vi "svx_Set Limits Interactively.vi"(7 "move upper or lower limit together":bool, 8 "error in":errorcluster, 10 "limits in":dbl[](array[numeric])=[0.0, 0.0, 0.0, 0.0, 0.0, 0.0, 0.0, 0.0, 0.0, 0.0, 0.0, 0.0, 0.0, 0.0, 0.0, 0.0, 0.0, 0.0, 0.0, 0.0], 11 "limit graph control refnum":refnum<vi>) -> (0 "error out":errorcluster, 2 "limits out":dbl[](array[numeric]), 3 "dup limit graph control refnum":refnum<vi>)   [LabVIEW 2017]
panel:
  out "limits graph":dbl[][](graph)
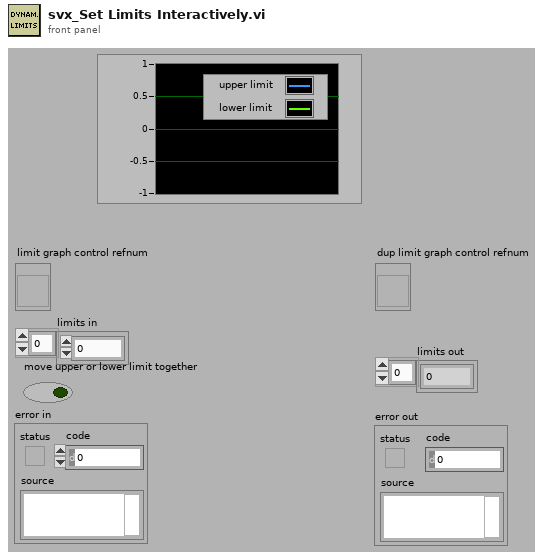
[diagram p1: front panel]
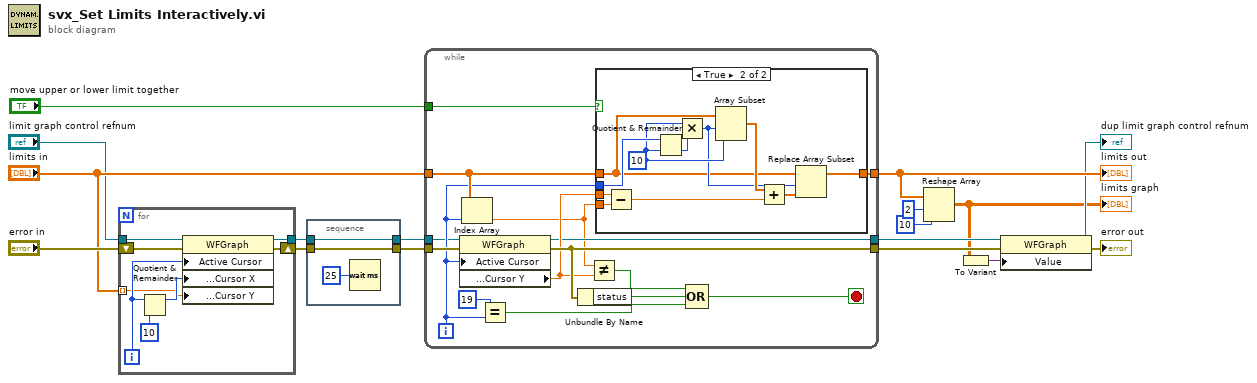
[diagram p0: block diagram]
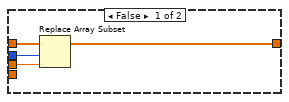
[diagram p2: hidden frame]
diagram:
  n1 = for {
    tunnel: "limits in" -> [w20] mode=indexing
    shift-right: [w21] -> w16
    shift-left: "error in" -> [w22]
    tunnel: "limit graph control refnum" -> [w19]
    tunnel: [w18] -> w9
    i -> [w24]
    n2 = Quotient & Remainder(x=w24, y=10) -> (x-y*floor(x/y)=w23:i32)  [unwired: 1 out]
    n3 = property class="WFGraph"(reference=w19, error in=w22, "Active Cursor"=w24, "Cursor.Cursor Position:Cursor X"=w23, "Cursor.Cursor Position:Cursor Y"=w20) -> (reference out=w18:refnum<vi>, error out=w21:errorcluster)
  }
  n4 = stacked-sequence {
    tunnel: w16 -> [w27]
    tunnel: [w27] -> w15
    tunnel: w9 -> [w26]
    tunnel: [w26] -> w8
    frame #0 {
      n5 = Wait (ms)(milliseconds to wait=u32 25) -> ()  [unwired: 1 out]
    }
  }
  n6 = while {
    tunnel: "limits in" -> [w37]
    tunnel: [w38] -> w13
    tunnel: w15 -> [w36]
    tunnel: [w35] -> w7
    tunnel: w8 -> [w32]
    tunnel: [w31] -> w6
    tunnel: "move upper or lower limit together" -> [w29]
    i -> [w34]
    stop <- w39 stop-if-true
    n7 = property class="WFGraph"(reference=w32, error in=w36, "Active Cursor"=w34) -> (reference out=w31:refnum<vi>, error out=w35:errorcluster, "Cursor.Cursor Position:Cursor Y"=w33:dbl)
    n8 = Index Array(array=w37, index=w34) -> (element=w30:dbl)
    n9 = Equal?(x=19, y=w34) -> (x = y?=w41:bool)
    n10 = Unbundle By Name(w35) -> ("status"=w43:bool)
    n11 = Not Equal?(x=w30, y=w33) -> (x != y?=w40:bool)
    n12 = case shown="True" w29 {
      tunnel: [w47 w49] -> w38
      tunnel: w37 -> [w46 w48]
      tunnel: w34 -> [w45 w55]
      tunnel: w33 -> [w44 w58]
      tunnel: w30 -> [_ w57]
      frame False {
        n13 = Replace Array Subset(array=w46, new element=w44, index=w45) -> (w47:dbl[])
      }
      frame True {
        w52 = 10 ("y")
        n14 = Subtract(x=w58, y=w57) -> (x-y=w56:dbl)
        n15 = Quotient & Remainder(x=w55, y=w52) -> (floor(x/y)=w54:i32)  [unwired: 1 out]
        n16 = Multiply(x=w52, y=w54) -> (x*y=w50:i32)
        n17 = Array Subset(array=w48, index=w50, length=w52) -> (w53:dbl[])
        n18 = Add(x=w53, y=w56) -> (x+y=w51:dbl[])
        n19 = Replace Array Subset(array=w48, new element=w51, index=w50) -> (w49:dbl[])
      }
    }
    n20 = Compound Arithmetic op=OR(w40, w43, w41) -> (w39:bool)
  }
  "limits out" <- w13
  n21 = Reshape Array(w13, 2 ("dimension size"), 10 ("dimension size")) -> (w2:dbl[][])
  "limits graph" <- w2
  n22 = To Variant(anything=w2) -> (Variant=w5:variant)
  n23 = property class="WFGraph"(reference=w6, error in=w7, "Value"=w5) -> (reference out=→"dup limit graph control refnum":refnum<vi>, error out=→"error out":errorcluster)
